vi "FT10_Unitherm Tester.vi"() -> ()   [LabVIEW 2015]
uses:
  Controls/QMH Fundamentals - Message Cluster.ctl
panel:
  in  "Reconnect":bool
  in  "Load (Ohms)":i32 max=6400 step=1
  in  "Set Load":bool
  in  "Clear Load":bool
  out "Status":bool[](array[boolean])
  in  "Get Status":bool
  in  "stop":bool
  out "Unitherm Connection empty?":bool
  out "error out":errorcluster
  out "UNITHERM Connection out":refnum<visa-resource-name>
  in  "error in (no error)":errorcluster
  in  "UNITHERM Connection in":refnum<visa-resource-name>
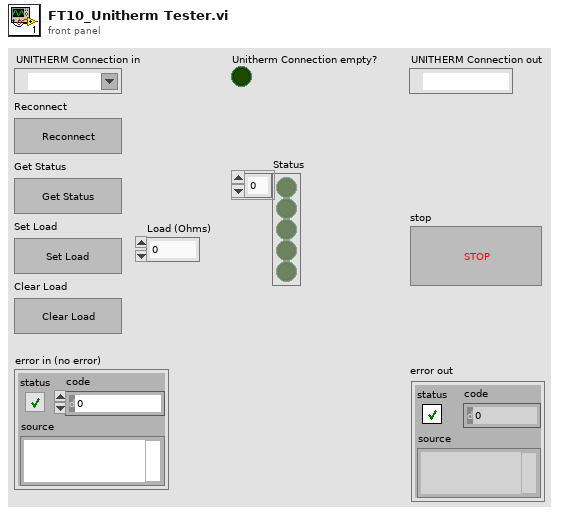
[diagram p1: front panel]
types:
  T1 = typedef "QMH Fundamentals - Message Cluster.ctl" = cluster{"Message":string, "Message Data":variant}
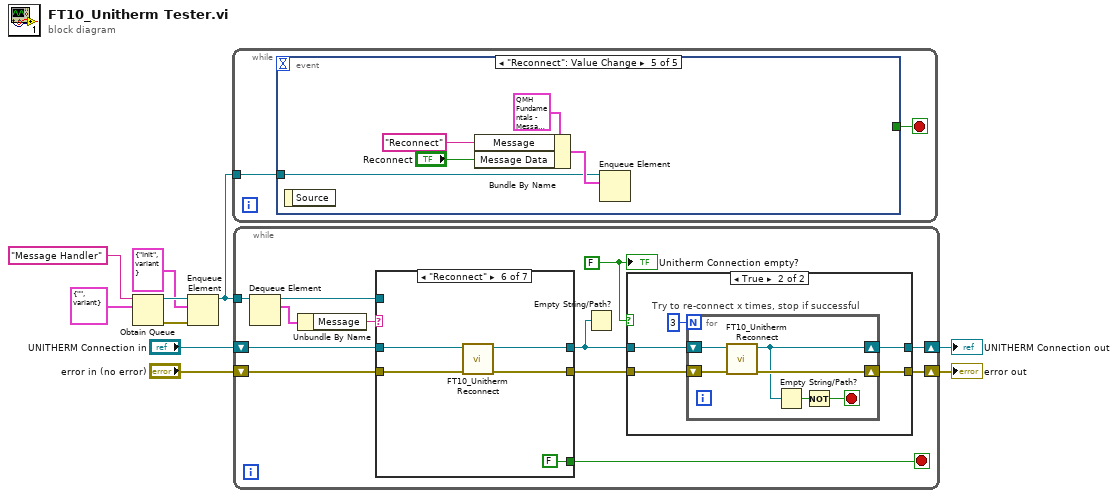
[diagram p0: block diagram]
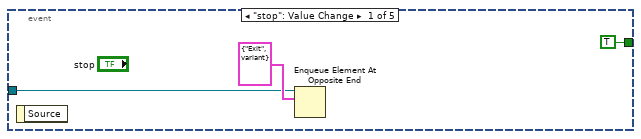
[diagram p2: hidden frame]
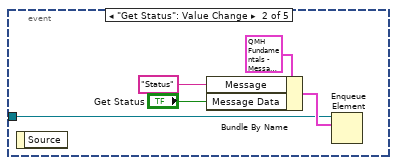
[diagram p3: hidden frame]
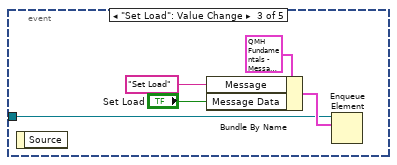
[diagram p4: hidden frame]
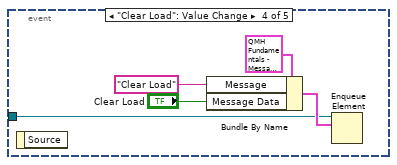
[diagram p5: hidden frame]
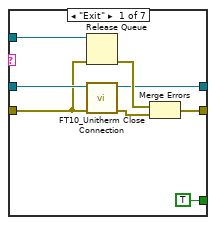
[diagram p6: hidden frame]
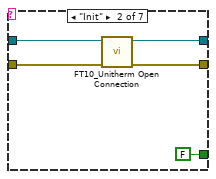
[diagram p7: hidden frame]
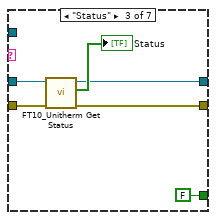
[diagram p8: hidden frame]
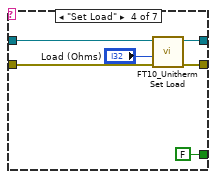
[diagram p9: hidden frame]
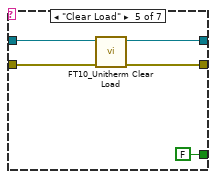
[diagram p10: hidden frame]
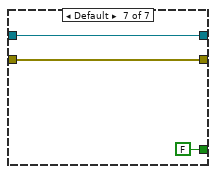
[diagram p11: hidden frame]
diagram:
  n1 = Obtain Queue(name (unnamed)="Message Handler", element data type=T1 {"Message"="", "Message Data"=variant} ("Message Cluster")) -> (queue out=w4:refnum<queue>, error out=w5:errorcluster)  [unwired: 3 in, 1 out]
  n2 = Enqueue Element(queue=w4, element=T1 {"Message"="Init", "Message Data"=variant}, error in (no error)=w5) -> (queue out=w1:refnum<queue>)  [unwired: 1 in, 2 out]
  n3 = while {
    tunnel: w1 -> [w12]
    stop <- w11 stop-if-true
    n4 = event shown="[4] \"Reconnect\": Value Change" {
      selector: _ -> [_ _ _ _ _]
      dyn-events: _ -> [_ _ _ _ _]
      timeout: _ -> [_ _ _ _ _]
      tunnel: w12 -> [w14 w16 w22 w27 w32]
      tunnel: [TRUE _ _ _ _] -> w11
      event "stop": Value Change {
        n5 = event-data() -> ()  [unwired: 1 in, 1 out]
        n6 = Enqueue Element At Opposite End(queue=w14, element=T1 {"Message"="Exit", "Message Data"=variant}) -> ()  [unwired: 2 in, 3 out]
      }
      event "Get Status": Value Change {
        n7 = event-data() -> ()  [unwired: 1 in, 1 out]
        n8 = Bundle By Name(cluster=T1 {"Message"="Fornax Connect/Disconnect", "Message Data"=variant} ("element"), "Message"="Status", "Message Data"="Get Status") -> (w20:T1)
        n9 = Enqueue Element(queue=w16, element=w20) -> ()  [unwired: 2 in, 3 out]
      }
      event "Set Load": Value Change {
        n10 = event-data() -> ()  [unwired: 1 in, 1 out]
        n11 = Bundle By Name(cluster=T1 {"Message"="Fornax Connect/Disconnect", "Message Data"=variant} ("element"), "Message"="Set Load", "Message Data"="Set Load") -> (w25:T1)
        n12 = Enqueue Element(queue=w22, element=w25) -> ()  [unwired: 2 in, 3 out]
      }
      event "Clear Load": Value Change {
        n13 = event-data() -> ()  [unwired: 1 in, 1 out]
        n14 = Bundle By Name(cluster=T1 {"Message"="Fornax Connect/Disconnect", "Message Data"=variant} ("element"), "Message"="Clear Load", "Message Data"="Clear Load") -> (w30:T1)
        n15 = Enqueue Element(queue=w27, element=w30) -> ()  [unwired: 2 in, 3 out]
      }
      event "Reconnect": Value Change {
        n16 = event-data() -> ()  [unwired: 1 in, 1 out]
        n17 = Bundle By Name(cluster=T1 {"Message"="Fornax Connect/Disconnect", "Message Data"=variant} ("element"), "Message"="Reconnect", "Message Data"="Reconnect") -> (w35:T1)
        n18 = Enqueue Element(queue=w32, element=w35) -> ()  [unwired: 2 in, 3 out]
      }
    }
  }
  n19 = while {
    shift-right: [w46] -> w8
    shift-left: "error in (no error)" -> [w39]
    shift-right: [w47] -> w9
    shift-left: "UNITHERM Connection in" -> [w41]
    tunnel: w1 -> [w44]
    stop <- w38 stop-if-true
    w36 = FALSE ("empty?")
    n20 = Dequeue Element(queue=w44) -> (queue out=w37:refnum<queue>, element=w45:T1)  [unwired: 2 in, 2 out]
    n21 = Unbundle By Name(w45) -> ("Message"=w43:string)
    n22 = case shown="\"Reconnect\"" w43 {
      tunnel: [w50 w59 w63 w68 w74 w80 w84] -> w42
      tunnel: w41 -> [w51 w60 w66 w71 w76 w81 w84]
      tunnel: [w53 w57 w62 w67 w73 w78 w83] -> w40
      tunnel: w39 -> [w48 w58 w65 w70 w75 w79 w83]
      tunnel: [TRUE FALSE FALSE FALSE FALSE FALSE FALSE] -> w38
      tunnel: w37 -> [w54 _ _ _ _ _ _]
      frame "Exit" {
        n23 = Release Queue(queue=w54, error in (no error)=w48) -> (error out=w52:errorcluster)  [unwired: 1 in, 2 out]
        n24 = call "FT10_Unitherm Close Connection.vi"("error in (no error)"=w48, "VISA Refnum in"=w51) -> ("error out"=w49:errorcluster, "VISA Refnum out"=w50:refnum<visa-resource-name>)  [unwired: 8 in]
        n25 = Merge Errors(w52, w49) -> (w53:errorcluster)
      }
      frame "Init" {
        n26 = call "FT10_Unitherm Open Connection.vi"("error in (no error)"=w58, "VISA Refnum in"=w60) -> ("error out"=w57:errorcluster, "VISA Refnum out"=w59:refnum<visa-resource-name>)  [unwired: 8 in]
      }
      frame "Status" {
        n27 = call "FT10_Unitherm Get Status.vi"("error in (no error)"=w65, "VISA Refnum in"=w66) -> ("error out"=w62:errorcluster, "Status"=→"Status":bool[], "VISA Refnum out"=w63:refnum<visa-resource-name>)  [unwired: 7 in]
      }
      frame "Set Load" {
        n28 = call "FT10_Unitherm Set Load.vi"("error in (no error)"=w70, "Load Impedance in"="Load (Ohms)", "VISA Refnum in"=w71) -> ("error out"=w67:errorcluster, "VISA Refnum out"=w68:refnum<visa-resource-name>)  [unwired: 5 in, 2 out]
      }
      frame "Clear Load" {
        n29 = call "FT10_Unitherm Clear Load.vi"("error in (no error)"=w75, "VISA Refnum in"=w76) -> ("error out"=w73:errorcluster, "VISA Refnum out"=w74:refnum<visa-resource-name>)  [unwired: 7 in, 1 out]
      }
      frame "Reconnect" {
        n30 = call "FT10_Unitherm Reconnect.vi"("error in (no error)"=w79, "VISA Refnum in"=w81) -> ("error out"=w78:errorcluster, "VISA Refnum out"=w80:refnum<visa-resource-name>)  [unwired: 8 in]
      }
      frame Default {
      }
    }
    n31 = Empty String/Path?(string/path=w42) -> ()  [unwired: 1 out]
    n32 = case shown="True" w36 {
      tunnel: w40 -> [w86 w92]
      tunnel: [w87 w91] -> w47
      tunnel: [w86 w90] -> w46
      tunnel: w42 -> [w87 w89]
      frame False {
      }
      frame True {
        n33 = for "Try to re-connect x times, stop if successful" {
          N: 3 -> [_]
          shift-right: [w97] -> w90
          shift-left: w92 -> [w98]
          shift-right: [w94] -> w91
          shift-left: w89 -> [w96]
          stop <- w93 stop-if-true
          n34 = call "FT10_Unitherm Reconnect.vi"("error in (no error)"=w98, "VISA Refnum in"=w96) -> ("error out"=w97:errorcluster, "VISA Refnum out"=w94:refnum<visa-resource-name>)  [unwired: 8 in]
          n35 = Empty String/Path?(string/path=w94) -> (empty?=w95:bool)
          n36 = Not(x=w95) -> (.not. x?=w93:bool)
        }
      }
    }
    "Unitherm Connection empty?" <- w36
  }
  "UNITHERM Connection out" <- w9
  "error out" <- w8
